vi "Day4Recurse.vi"(7 "Direction":T1, 8 "Character Array":string[][](array[string]), 9 "Letter":string, 10 "YIndex":i32, 11 "XIndex":i32) -> (3 "XMASCount":i64)   [LabVIEW 2024]
uses:
  Day4Direction.ctl
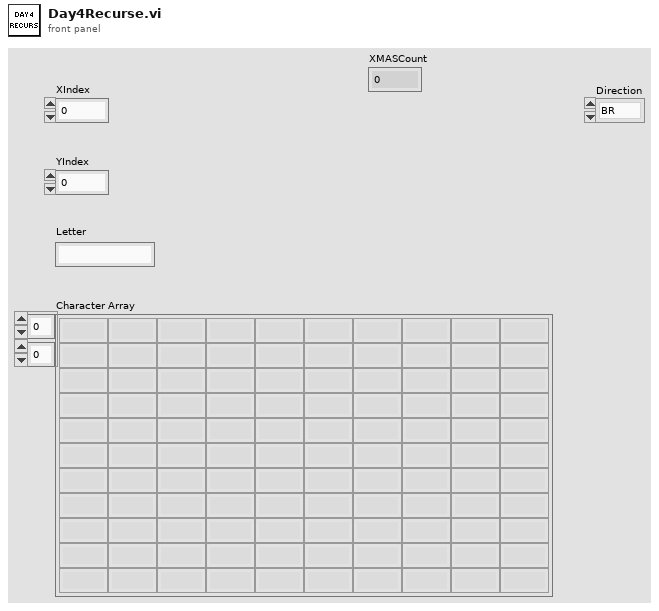
[diagram p1: front panel]
types:
  T1 = typedef "Day4Direction.ctl" = enum16{"BR", "BL", "B", "R", "L", "UR", "UL", "U"}
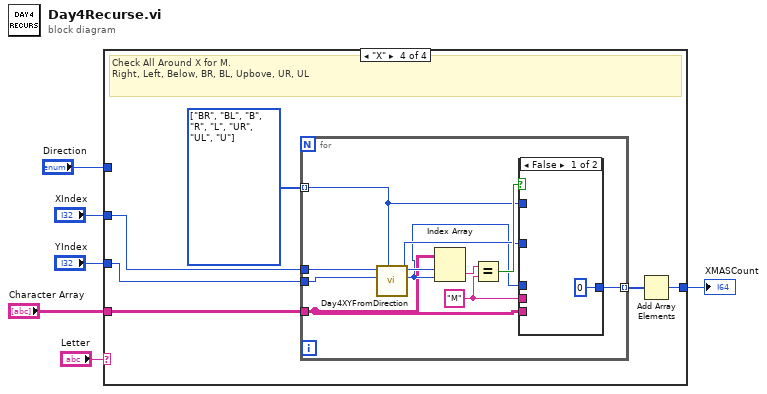
[diagram p0: block diagram]
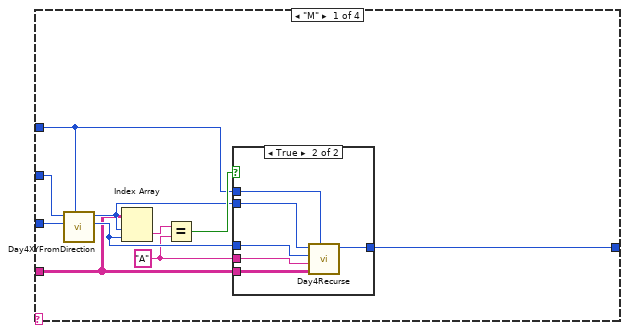
[diagram p2: hidden frame]
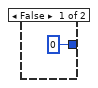
[diagram p3: hidden frame]
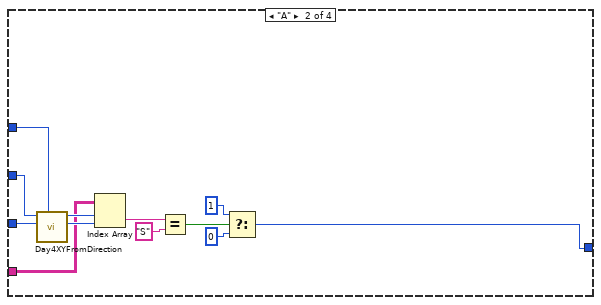
[diagram p4: hidden frame]
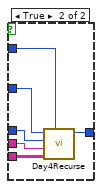
[diagram p6: hidden frame]
diagram:
  n1 = case shown="\"X\"" "Letter" {
    tunnel: "XIndex" -> [w16 w35 _ w39]
    tunnel: "Character Array" -> [w9 w29 _ w41]
    tunnel: "YIndex" -> [w15 w34 _ w38]
    tunnel: "Direction" -> [w8 w28 _ _]
    tunnel: [w7 w24 _ w37] -> w1
    frame "M" {
      w10 = "A"
      n2 = call "Day4XYFromDirection.vi"("Direction"=w8, "YIndex"=w15, "XIndex"=w16) -> ("NewY"=w11:i32, "NewX"=w12:i32)  [unwired: 7 in]
      n3 = Index Array(array=w9, index (row)=w12, index (col)=w11) -> (element=w14:string)
      n4 = Equal?(x=w14, y=w10) -> (x = y?=w13:bool)
      n5 = case shown="True" w13 {
        tunnel: w12 -> [_ w23]
        tunnel: w11 -> [_ w22]
        tunnel: w10 -> [_ w21]
        tunnel: w9 -> [_ w20]
        tunnel: w8 -> [_ w19]
        tunnel: [i64 0 ("XMASCount") w18] -> w7
        frame False {
        }
        frame True {
          n6 = call "Day4Recurse.vi"("Direction"=w19, "Character Array"=w20, "Letter"=w21, "YIndex"=w22, "XIndex"=w23) -> ("XMASCount"=w18:i64)  [unwired: 6 in]
        }
      }
    }
    frame "A" {
      n7 = call "Day4XYFromDirection.vi"("Direction"=w28, "YIndex"=w34, "XIndex"=w35) -> ("NewY"=w31:i32, "NewX"=w32:i32)  [unwired: 7 in]
      n8 = Index Array(array=w29, index (row)=w32, index (col)=w31) -> (element=w33:string)
      n9 = Equal?(x=w33, y="S") -> (x = y?=w27:bool)
      n10 = Select(t=i64 1, s=w27, f=i64 0) -> (s? t:f=w24:i64)
    }
    frame Default {
    }
    frame "X" {
      w40 = T1[] [enum."BR", enum."BL", enum."B", enum."R", enum."L", enum."UR", enum."UL", enum."U"] items=["BR", "BL", "B", "R", "L", "UR", "UL", "U"]
      # "Check All Around X for M.\nRight, Left, Below, BR, BL, Upbove, UR, UL"
      n11 = for {
        tunnel: w41 -> [w43]
        tunnel: w40 -> [w44] mode=indexing
        tunnel: w39 -> [w48]
        tunnel: w38 -> [w47]
        tunnel: [w42] -> w36 mode=indexing
        w50 = "M"
        n12 = call "Day4XYFromDirection.vi"("Direction"=w44, "YIndex"=w47, "XIndex"=w48) -> ("NewY"=w45:i32, "NewX"=w46:i32)  [unwired: 7 in]
        n13 = Index Array(array=w43, index (row)=w46, index (col)=w45) -> (element=w51:string)
        n14 = Equal?(x=w51, y=w50) -> (x = y?=w49:bool)
        n15 = case shown="False" w49 {
          tunnel: w50 -> [_ w58]
          tunnel: w44 -> [_ w57]
          tunnel: w46 -> [_ w56]
          tunnel: w45 -> [_ w55]
          tunnel: w43 -> [_ w54]
          tunnel: [i64 0 ("XMASCount") w53] -> w42
          frame False {
          }
          frame True {
            n16 = call "Day4Recurse.vi"("Direction"=w57, "Character Array"=w54, "Letter"=w58, "YIndex"=w55, "XIndex"=w56) -> ("XMASCount"=w53:i64)  [unwired: 6 in]
          }
        }
      }
      n17 = Add Array Elements(numeric array=w36) -> (sum=w37:i64)
    }
  }
  "XMASCount" <- w1
